vi "Bai3_3_C2.vi"() -> ()   [LabVIEW 2019]
panel:
  out "error out":errorcluster
  in  "error in":errorcluster
  in  "Stop":bool=TRUE
  in  "Lines to Write":u16(ring) items=["0 - 7", "8 - 15", "16 - 23"]
  in  "Device Name":tag="Dev8"
  in  "stop":bool
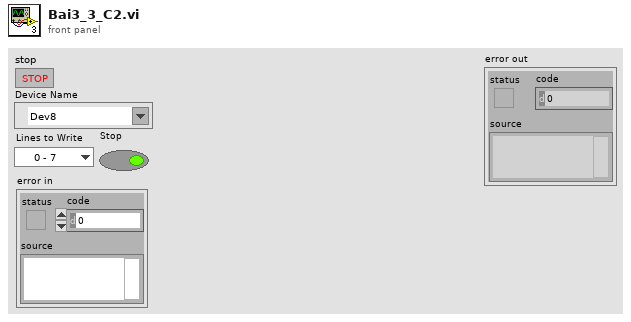
[diagram p1: front panel]
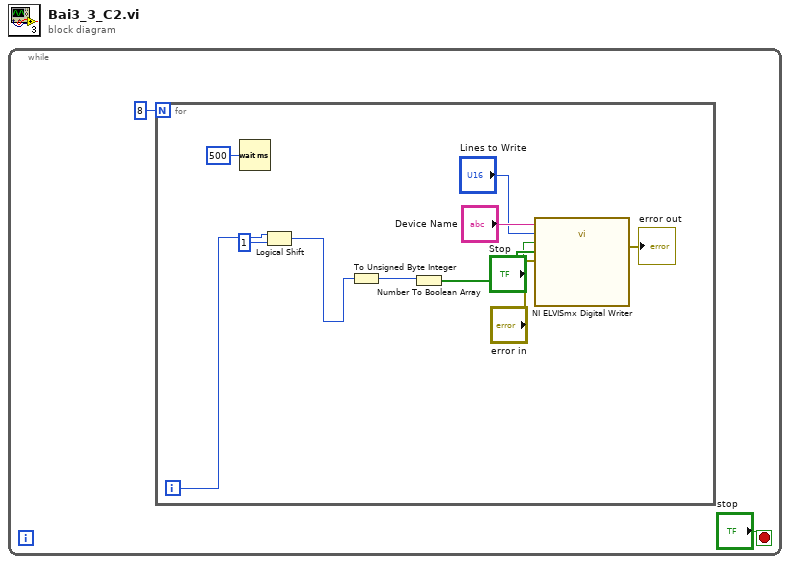
[diagram p0: block diagram]
diagram:
  n1 = while {
    stop <- "stop" stop-if-true
    n2 = for {
      N: 8 -> [_]
      i -> [w10]
      n3 = Wait (ms)(milliseconds to wait=u32 500) -> ()  [unwired: 1 out]
      n4 = Logical Shift(y=w10, x=1) -> (x << y=w13:i32)
      n5 = To Unsigned Byte Integer(number=w13) -> (unsigned 8bit integer=w12:u8)
      n6 = Number To Boolean Array(number=w12) -> (Boolean array=w11:bool[])
      n7 = call "NI ELVISmx Digital Writer"("Device Name"="Device Name", "Lines to Write"="Lines to Write", "Stop"="Stop", "DO Lines"=w11, "error in"="error in") -> ("error out"=→"error out":errorcluster)  [unwired: 14 in]
    }
  }
